vi "SetPerformanceGlobals.vi"(8 "error in (no error)":errorcluster, 10 "Performance globals":T1, 11 "SM1000-control in":T2) -> (0 "error out":errorcluster, 3 "SM1000-control out":T2)   [LabVIEW 2013, in "MaterialCharacterization.lvlib" / "MC-SM1000.lvclass"]
doc: "Set factors to alter the run-time performance of the system.\n\nThese factors alter the specified marking properties without the need for changing the job. These values are volatile and will not be valid if the EC1000 is reset.\n\nCommand: <\"SetPerformanceGlobals\">,<mark-speed-adjust>,<laser-power-adjust>,<pulse-width-adjust>,<pulse-period-adjust>,<orientation>,<X-offset>,<Y-offset>,<Z-offset> or 14, <mark-speed-adjust>,<laser-power-adjust>,<pulse-width-adjust>,<pulse-period-adjust>,<orientation>,<X-offset>,<Y-offset>,<Z-offset>\nReturns: \"0\""
uses:
  MC-SM1000.lvclass
  Object-reference.ctl
  Performance-globals.ctl
  MC-SM1000.lvclass/MC-SM1000.ctl
  Custom-errors.ctl
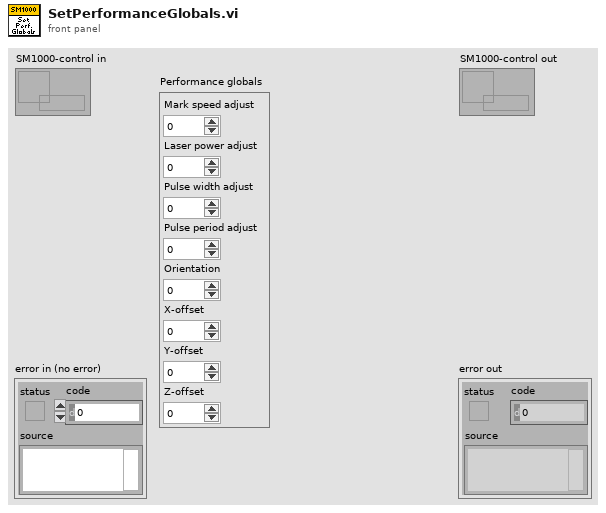
[diagram p1: front panel]
types:
  T1 = typedef "MaterialCharacterization.lvlib/MC-SM1000.lvclass/Performance-globals.ctl" = cluster{"Mark speed adjust":dbl, "Laser power adjust":dbl, "Pulse width adjust":dbl, "Pulse period adjust":dbl, "Orientation":i32, "X-offset":i32, "Y-offset":i32, "Z-offset":i32}
  T2 = typedef "MaterialCharacterization.lvlib/MC-SM1000.lvclass/Object-reference.ctl" = refnum<data-value>
  T3 = typedef "MaterialCharacterization.lvlib/MC-SM1000.lvclass/Custom-errors.ctl" = enum16{"No error", "Not implemented", "Command not recognized", "Invalid input", "No connection", "Timeout", "Resource not loaded"}
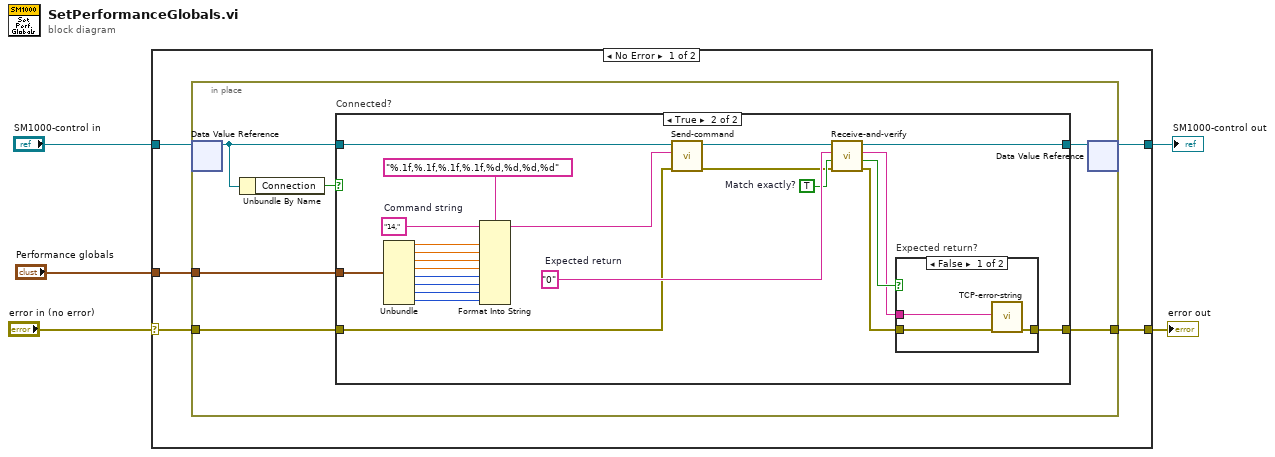
[diagram p0: block diagram]
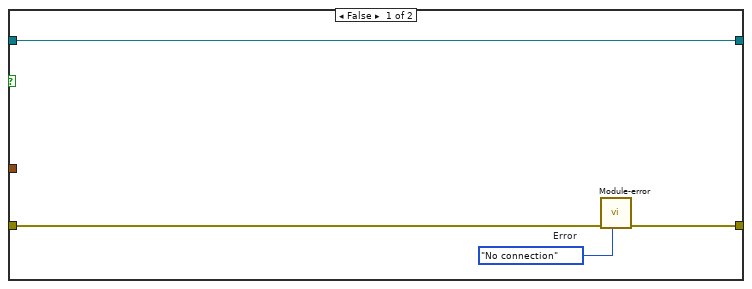
[diagram p2: hidden frame]
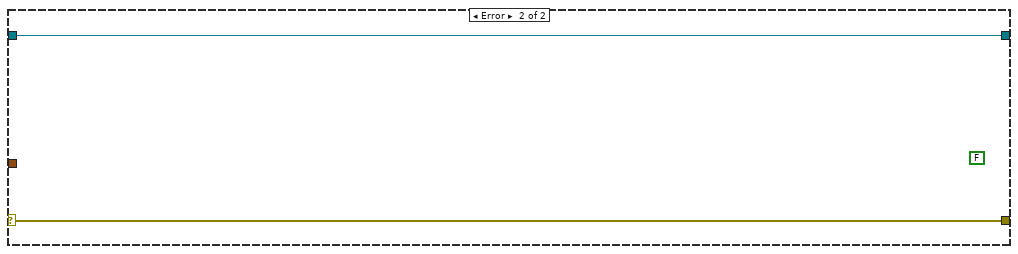
[diagram p4: hidden frame]
diagram:
  n1 = case shown="No Error" "error in (no error)" {
    selector: "error in (no error)" -> [w8 w49]
    tunnel: [w7 w49] -> w4
    tunnel: [w9 w48] -> w2
    tunnel: "SM1000-control in" -> [w10 w48]
    tunnel: "Performance globals" -> [w6 _]
    frame No Error {
      n2 = in-place {
        in-place-border: w8 -> [w16]
        in-place-border: [w13] -> w7
        in-place-border: w6 -> [w11]
        n3 = in-place-dvr #1(w10) -> (w14:refnum<class "MC-SM1000.lvclass">)  [unwired: 1 out]
        n4 = Unbundle By Name(w14) -> ("Connection"=w15:bool)
        n5 = case "Connected?" shown="True" w15 {
          tunnel: w16 -> [w20 w36]
          tunnel: w14 -> [w18 w43]
          tunnel: [w19 w34] -> w13
          tunnel: [w18 w33] -> w12
          tunnel: w11 -> [_ w31]
          frame False {
            w17 = Custom-errors."No connection"  # Error
            n6 = call "Module-error.vi"("Error"=w17, "error in (no error)"=w20) -> ("error out"=w19:errorcluster)  [unwired: 9 in]
          }
          frame True {
            w40 = TRUE  # Match exactly?
            w41 = "0"  # Expected return
            w32 = "14,"  # Command string
            n7 = Unbundle(w31) -> ("Mark speed adjust"=w30:dbl, "Laser power adjust"=w29:dbl, "Pulse width adjust"=w28:dbl, "Pulse period adjust"=w27:dbl, "Orientation"=w26:i32, "X-offset"=w25:i32, "Y-offset"=w24:i32, "Z-offset"=w23:i32)
            n8 = Format Into String(format string="%.1f,%.1f,%.1f,%.1f,%d,%d,%d,%d", initial string=w32, w30, w29, w28, w27, w26, w25, w24, w23) -> (resulting string=w21:string)  [unwired: 1 in, 1 out]
            n9 = call "Send-command.vi"("error in (no error)"=w36, "Command string"=w21, "SM1000-control in"=w43) -> ("error out"=w39:errorcluster, "SM1000-control out"=w42:refnum<class "MC-SM1000.lvclass">)  [unwired: 7 in]
            n10 = call "Receive-and-verify.vi"("error in (no error)"=w39, "Match exactly?"=w40, "Expected return string"=w41, "SM1000-control in"=w42) -> ("error out"=w35:errorcluster, "Verified?"=w38:bool, "Return string"=w37:string, "SM1000-control out"=w33:refnum<class "MC-SM1000.lvclass">)  [unwired: 4 in]
            n11 = case "Expected return?" shown="False" w38 {
              tunnel: w37 -> [w46 _]
              tunnel: w35 -> [w45 w47]
              tunnel: [w44 w47] -> w34
              frame False {
                n12 = call "TCP-error-string.vi"("error in (no error)"=w45, "Retun code"=w46) -> ("error out"=w44:errorcluster)  [unwired: 9 in]
              }
              frame True {
              }
            }
          }
        }
        n13 = in-place-dvr #1(w12) -> (w9:T2)  [unwired: 1 out]
      }
    }
    frame Error {
      (unwired) FALSE
    }
  }
  "error out" <- w4
  "SM1000-control out" <- w2
